vi "Read Active Cell Position Top.vi"(8 "error in (no error)":errorcluster, 11 "Table.lvclass in":refnum<class "Table.lvclass">) -> (0 "error out":errorcluster, 2 "ActiveCellPosTop":i32, 3 "Table.lvclass out":refnum<class "Table.lvclass">)   [LabVIEW 2015, in "Table.lvclass"]
uses:
  Table.lvclass
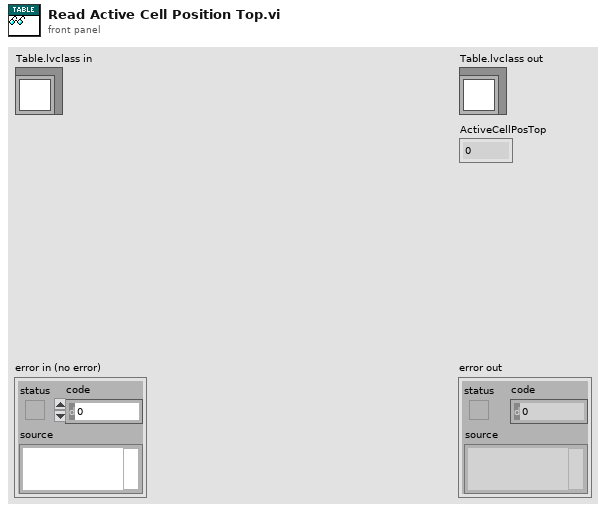
[diagram p1: front panel]
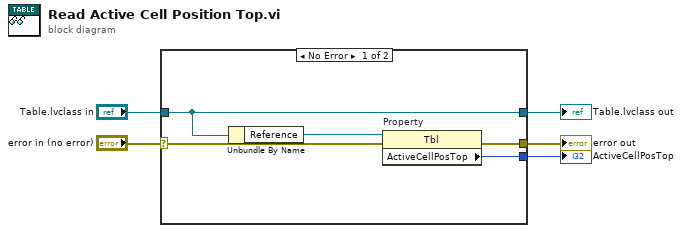
[diagram p0: block diagram]
diagram:
  n1 = case shown="No Error" "error in (no error)" {
    selector: "error in (no error)" -> [w6 w12]
    tunnel: [w9 w12] -> w4
    tunnel: [w8 w11] -> w2
    tunnel: "Table.lvclass in" -> [w8 w11]
    tunnel: [w10 _] -> w1
    frame No Error {
      n2 = Unbundle By Name(w8) -> ("Reference"=w7:refnum<vi>)
      n3 = property on="Property" class="Tbl"(reference=w7, error in=w6) -> (error out=w9:errorcluster, "ActiveCellPosTop"=w10:i32)  [unwired: 1 out]
    }
    frame Error {
    }
  }
  "error out" <- w4
  "Table.lvclass out" <- w2
  "ActiveCellPosTop" <- w1
